vi "Launch_VI_Asynchronously.vi"(8 "error in (no error)":errorcluster, 9 "Value":variant[](array[variant]), 10 "Control Names":string[](array[string]), 11 "vi path":path) -> (0 "error out":errorcluster)   [LabVIEW 2020]
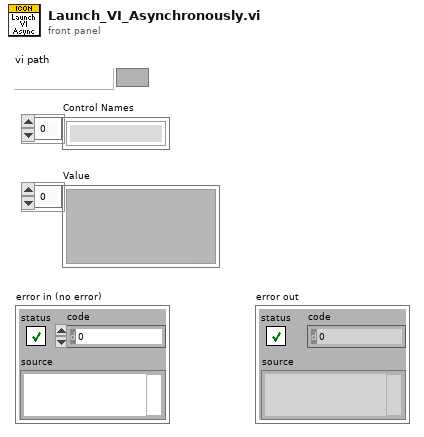
[diagram p1: front panel]
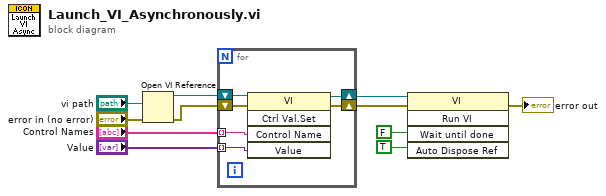
[diagram p0: block diagram]
diagram:
  n1 = Open VI Reference(vi path="vi path", error in (no error)="error in (no error)") -> (vi reference=w6:refnum<vi>, error out=w5:errorcluster)  [unwired: 4 out]
  n2 = for {
    shift-right: [w15] -> w4
    shift-left: w6 -> [w17]
    shift-right: [w14] -> w3
    shift-left: w5 -> [w16]
    tunnel: "Control Names" -> [w13] mode=indexing
    tunnel: "Value" -> [w12] mode=indexing
    n3 = invoke class="VI" method="Ctrl Val.Set"(reference=w17, error in=w16, "Control Name"=w13, "Value"=w12) -> (reference out=w15:refnum<vi>, error out=w14:errorcluster)  [unwired: 1 in, 3 out]
  }
  n4 = invoke class="VI" method="Run VI"(reference=w4, error in=w3, "Wait until done"=FALSE ("Wait Until Done"), "Auto Dispose Ref"=TRUE ("Auto Dispose Reference")) -> (error out=→"error out":errorcluster)  [unwired: 1 in, 4 out]
